vi "LVClass_HasoSlopes Get Intensity.vi"(0 "HasoSlopes in":refnum<class "HasoSlopes.lvclass">, 11 "error in (no error)":errorcluster) -> (4 "HasoSlopes out":refnum<class "HasoSlopes.lvclass">, 6 "Intensity":i32[][](array[numeric]), 15 "error out":errorcluster)   [LabVIEW 2020, in "HasoSlopes.lvclass"]
doc: "HasoSlopes intensity buffer getter.\n\n--------------------------------------------------------------------------------\n\n<B>HasoSlopesIn </B> : HasoSlopes object.\n<B>HasoSlopesOut </B> : HasoSlopes object.\n<B>intensity </B> : 2D Intensity buffer\n<B>ErrorIn </B> : Error\n<B>ErrorOut </B> : Error\n\n--------------------------------------------------------------------------------"
uses:
  HasoSlopes.lvclass
  HasoSlopes.lvclass/HasoSlopes.ctl
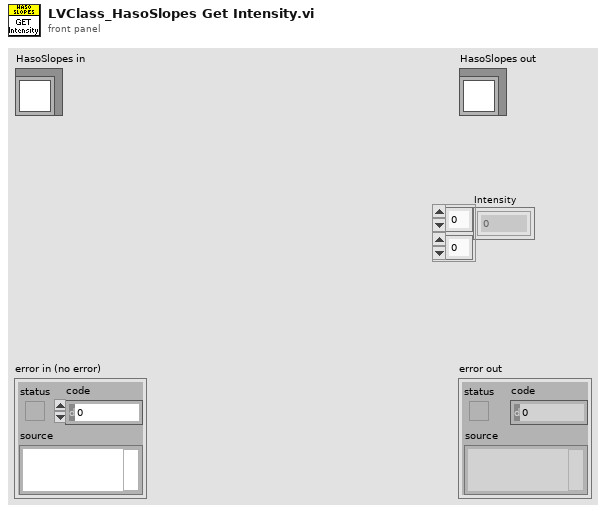
[diagram p1: front panel]
types:
  T1 = typedef "Point2D.ctl" = cluster{"X":u32, "Y":u32}
  T2 = typedef "Point2Df.ctl" = cluster{"X":sgl, "Y":sgl}
  T3 = typedef "ClassID.ctl" = i64
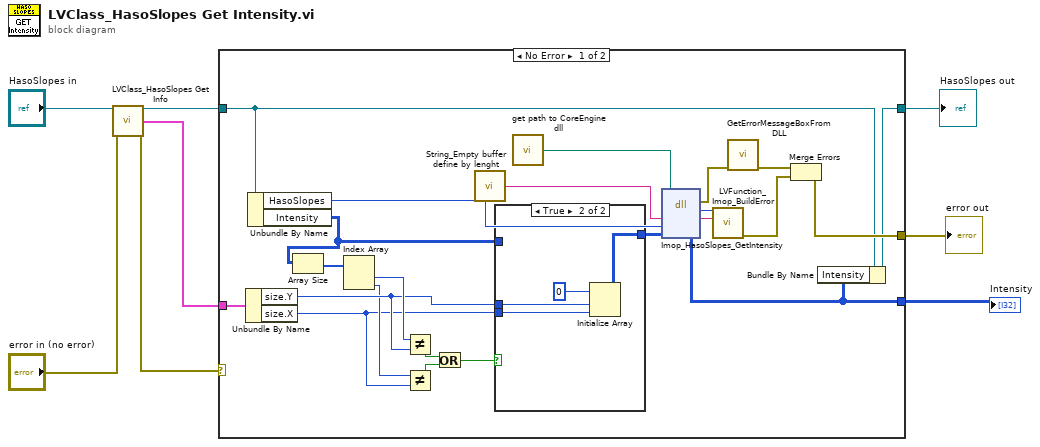
[diagram p0: block diagram]
diagram:
  n1 = call "LVClass_HasoSlopes Get Info.vi"("HasoSlopes in"="HasoSlopes in", "error in (no error)"="error in (no error)") -> ("HasoSlopes out"=w4:refnum<class "HasoSlopes.lvclass">, "dimension"=w1:cluster{"size":T1, "step":T2}, "error out"=w3:errorcluster)  [unwired: 9 in, 2 out]
  n2 = case shown="No Error" w3 {
    selector: w3 -> [_ w38]
    tunnel: [w21 w38] -> w8
    tunnel: [w18 w37] -> w7
    tunnel: w4 -> [w19 w37]
    tunnel: [w20 _] -> w6
    tunnel: w1 -> [w24 _]
    frame No Error {
      n3 = Unbundle By Name(w24) -> ("size.Y"=w15:u32, "size.X"=w13:u32)
      n4 = Unbundle By Name(w19) -> ("HasoSlopes"=w28:T3, "Intensity"=w12:i32[][])
      n5 = Array Size(array=w12) -> (size(s)=w17:i32[])
      n6 = Index Array(array=w17) -> (element #1=w16:i32, element #2=w14:i32)  [unwired: 2 in]
      n7 = Not Equal?(x=w16, y=w15) -> (x != y?=w11:bool)
      n8 = Not Equal?(x=w14, y=w13) -> (x != y?=w10:bool)
      n9 = Or(x=w11, y=w10) -> (x .or. y?=w9:bool)
      n10 = call "String_Empty buffer define by lenght.vi"() -> ("Empty buffer"=w31:string)  [unwired: 1 in]
      n11 = case shown="True" w9 {
        tunnel: [w32 w33] -> w25
        tunnel: w15 -> [_ w35]
        tunnel: w13 -> [_ w34]
        tunnel: w12 -> [w32 _]
        frame False {
        }
        frame True {
          n12 = Initialize Array(0, w35, w34) -> (w33:i32[][])
        }
      }
      n13 = call "get path to CoreEngine dll.vi"() -> ("path to wavekit library"=w27:path)  [unwired: 14 in, 1 out]
      n14 = dll-call lib="D:/soft/HASO_v3/SVN_trunk/ImOpCoreEngine4_LV2011/DLLs/c_interface_vc100.dll" fn="Imop_HasoSlopes_GetIntensity"(path in=w27, "message"=w31, "objet"=w28, "Intensity"=w25) -> (error out=w26:errorcluster, "return type"=w29:i32, "message"=w30:string, "Intensity"=w20:i32[][])  [unwired: 3 in, 1 out]
      n15 = call "LVFunction_Imop_BuildError.vi"("code"=w29, "String to Prepend to source (\"\")"=w30) -> ("error out"=w22:errorcluster)  [unwired: 13 in]
      n16 = call "GetErrorMessageBoxFromDLL.vi"("error IN"=w26) -> ("error OUT"=w23:errorcluster)  [unwired: 10 in]
      n17 = Merge Errors(w23, w22) -> (w21:errorcluster)
      n18 = Bundle By Name(cluster=w19, "Intensity"=w20) -> (w18:refnum<class "HasoSlopes.lvclass">)
    }
    frame Error {
    }
  }
  "error out" <- w8
  "HasoSlopes out" <- w7
  "Intensity" <- w6
